vi "Extract Image Data X.vi"(6 "Averaged Values":dbl[][](array[numeric]), 7 "Filter Size":i32=5, 9 "Array":dbl[](array[numeric]), 10 "Bounding Box":cluster{dbl, dbl, dbl, dbl, dbl}) -> (2 "Centerpoint":cluster{dbl, dbl})   [LabVIEW 2018]
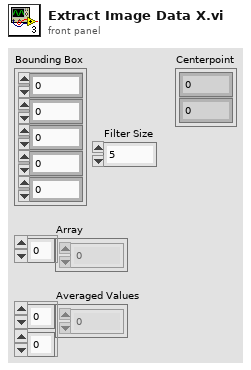
[diagram p1: front panel]
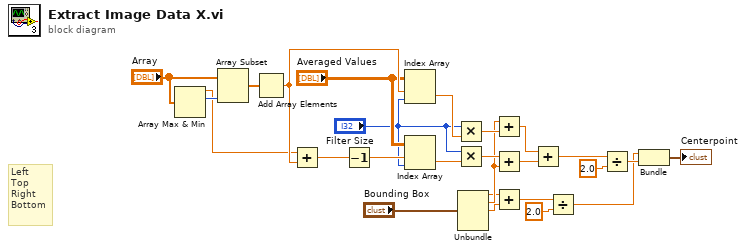
[diagram p0: block diagram]
diagram:
  # "Left\nTop\nRight\nBottom"
  n1 = Array Max & Min(array="Array") -> (max value=w17:dbl, max index (indices)=w21:i32)  [unwired: 2 out]
  n2 = Array Subset(array="Array", length=w21) -> (w15:dbl[])  [unwired: 1 in]
  n3 = Add Array Elements(numeric array=w15) -> (sum=w18:dbl)
  n4 = Add(x=w17, y=w18) -> (x+y=w19:dbl)
  n5 = Decrement(x=w19) -> (x-1=w20:dbl)
  n6 = Index Array(array="Averaged Values", index (row)=w18, index (col)="Filter Size") -> (element=w24:dbl)
  n7 = Index Array(array="Averaged Values", index (row)=w20, index (col)="Filter Size") -> (element=w25:dbl)
  n8 = Multiply(x="Filter Size", y=w24) -> (x*y=w22:dbl)
  n9 = Multiply(x="Filter Size", y=w25) -> (x*y=w23:dbl)
  n10 = Unbundle("Bounding Box") -> (w2:dbl, w12:dbl, w3:dbl)  [unwired: 2 out]
  n11 = Add(x=w12, y=w22) -> (x+y=w7:dbl)
  n12 = Add(x=w23, y=w12) -> (x+y=w6:dbl)
  n13 = Add(x=w2, y=w3) -> (x+y=w8:dbl)
  n14 = Add(x=w7, y=w6) -> (x+y=w11:dbl)
  n15 = Divide(x=w8, y=2.0) -> (x/y=w4:dbl)
  n16 = Divide(x=w11, y=2.0) -> (x/y=w5:dbl)
  n17 = Bundle(w4, w5) -> (→"Centerpoint":cluster{dbl, dbl})  [unwired: 1 in]
